vi "Input Quantities.vi"() -> ()   [LabVIEW 2013]
uses:
  qwtblvlib/TD Quantity.ctl
  TD Input Quantities qeue values.ctl
  <vilib>/Analysis/Matrix/Datatypes/RealMatrix.ctl
  globals.vi
  <vilib>/Utility/xml.llb/Write to XML File(string).vi
  <vilib>/Utility/xml.llb/Read From XML File(string).vi
  <vilib>/Utility/file.llb/Read From Spreadsheet File (DBL).vi
  <vilib>/Analysis/Matrix/Numeric/Conversions/Matrix To Array - RM.vi
  <vilib>/Analysis/Matrix/NI_Matrix.lvlib
  qwtblvlib/QWTBLVLib.lvlib
panel:
  in  "qeue cases":T1=enum."update list of quantities"
  out "current Q index":i32 min=0
  in  "r-randomize":bool
  in  "corr-default":bool
  in  "dof-fill":bool
  in  "uncertainty-fill":bool
  in  "value-load CSV":bool
  in  "hide this panel":bool
  in  "import data":bool
  in  "generate wvfrm":bool
  in  "Q":T2={"Name"="", "Value"=[[1.0]], "Uncertainty"=[[1.0]], "Degrees of Freedom"=[[10.0]], "Correlation"=[[10.0]], "Randomized uncertainty"=[[10.0]]} caption="Selected Quantity"
  in  "load all":bool
  in  "save all":bool
  in  "Q list":i32(listbox) caption="List of\nInput Quantities"
  in  "remove Q":bool
  in  "add Q":bool
  in  "rand-clear":bool
  in  "corr-clear":bool
  in  "dof-clear":bool
  in  "uncertainty-clear":bool
  in  "value-clear":bool
  # "Input Quantities"
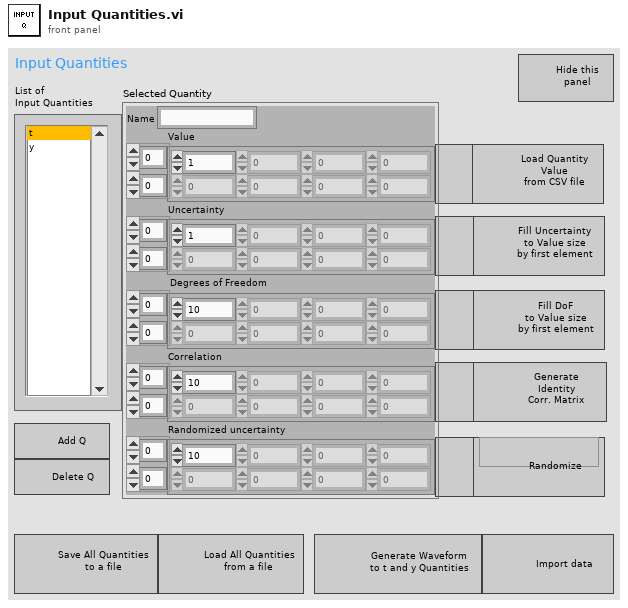
[diagram p1: front panel]
types:
  T1 = typedef "TD Input Quantities qeue values.ctl" = enum16{"hide VI", "current Q to datain", "update list of quantities", "show current quantity", "quit"}
  T2 = typedef "QWTBLVLib.lvlib/TD Quantity.ctl" = cluster{"Name":string, "Value":dbl[][], "Uncertainty":dbl[][], "Degrees of Freedom":dbl[][], "Correlation":dbl[][], "Randomized uncertainty":dbl[][]}
  T3 = enum32{"Invalid", "Standard", "Closed", "Hidden", "Minimized", "Maximized"}
  T4 = enum8{"Enabled", "Disabled", "Disabled and Grayed Out"}
  T5 = cluster{"Name":string, "Value":dbl[][], "Uncertainty":dbl[][], "Degrees of\nFreedom":dbl[][], "Correlation":dbl[][], "Randomized uncertainty":dbl[][]}
  T6 = typedef "NI_Matrix.lvlib/RealMatrix.ctl" = dbl[][]
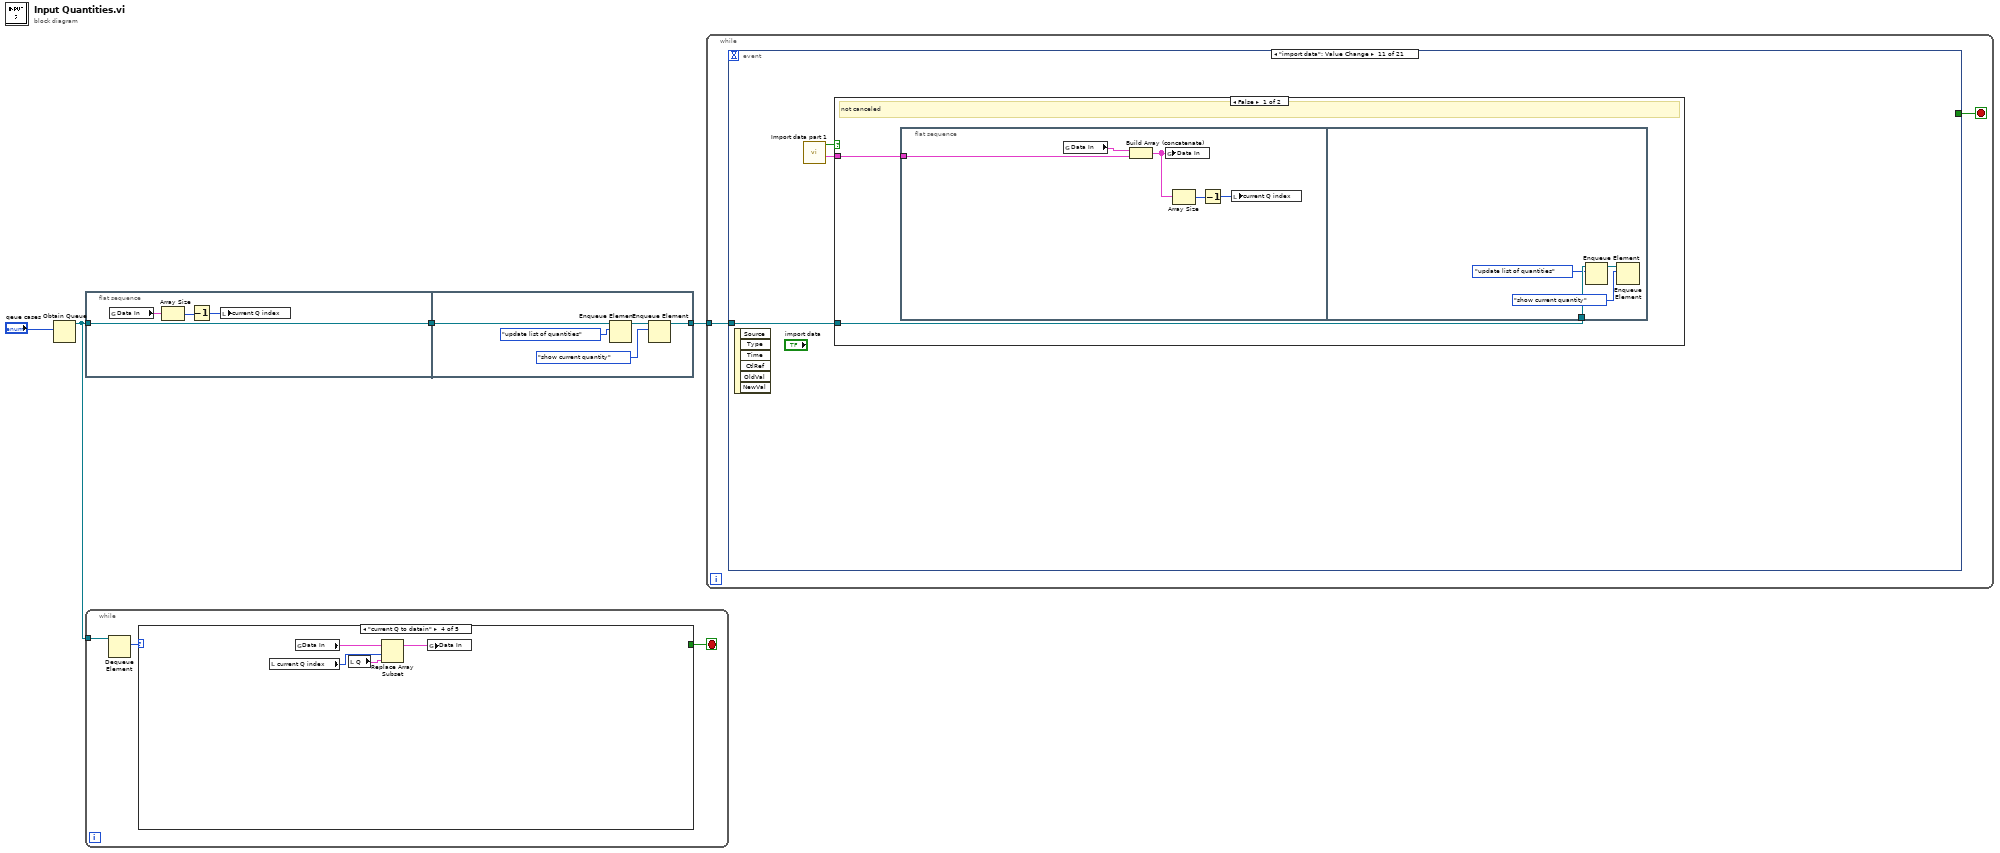
[diagram p0: block diagram]
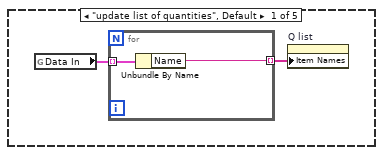
[diagram p2: hidden frame]
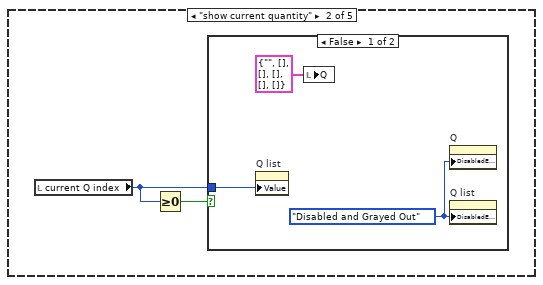
[diagram p3: hidden frame]
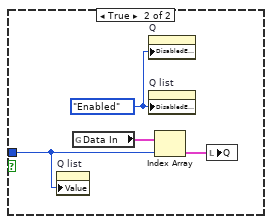
[diagram p4: hidden frame]
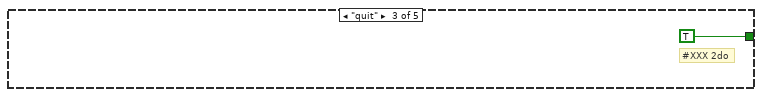
[diagram p5: hidden frame]
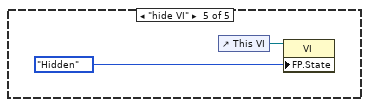
[diagram p6: hidden frame]
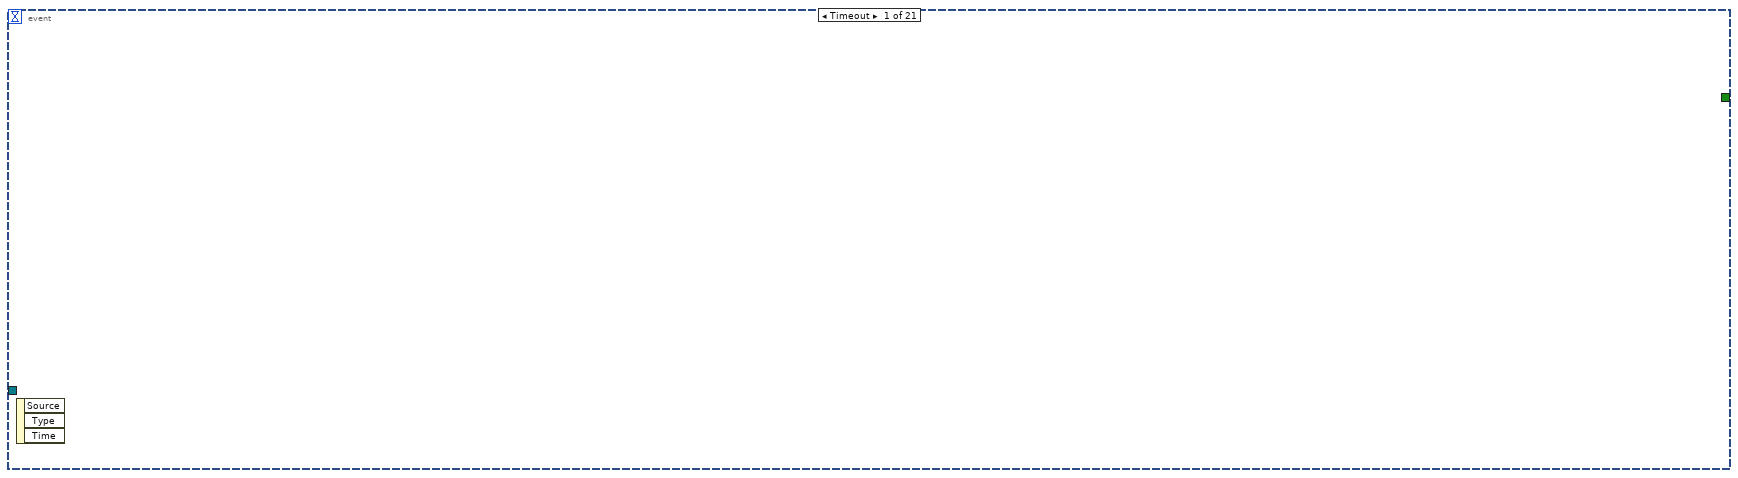
[diagram p7: hidden frame]
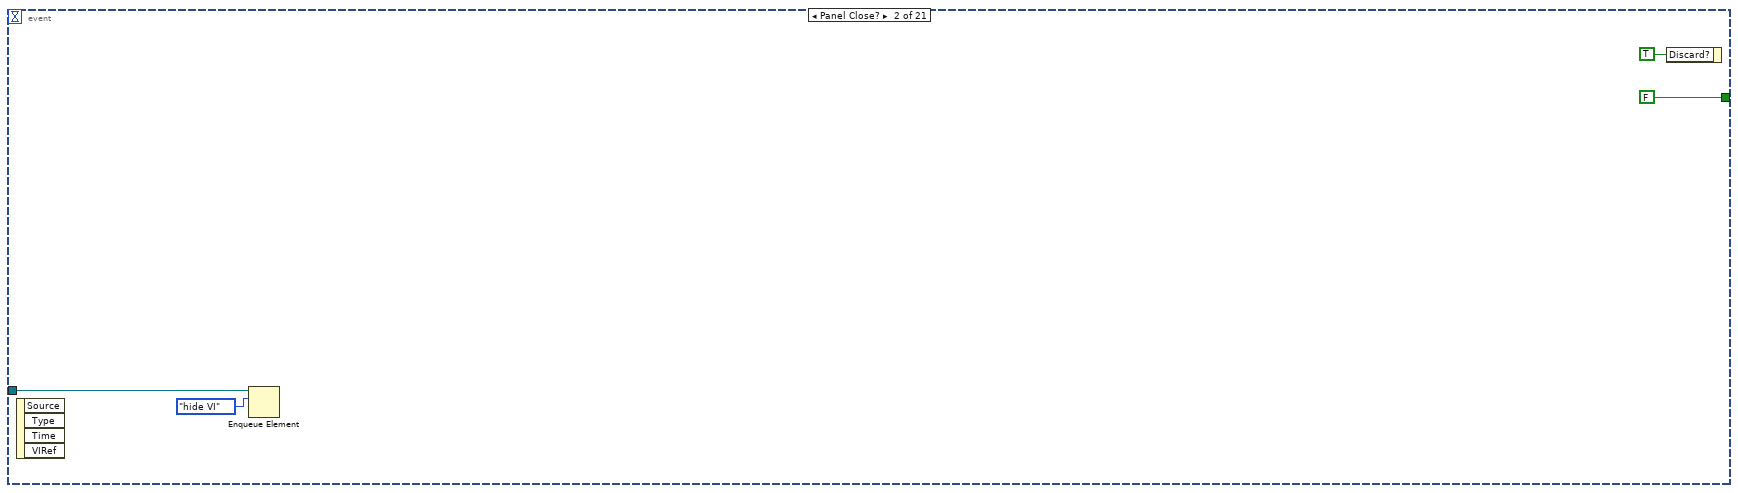
[diagram p8: hidden frame]
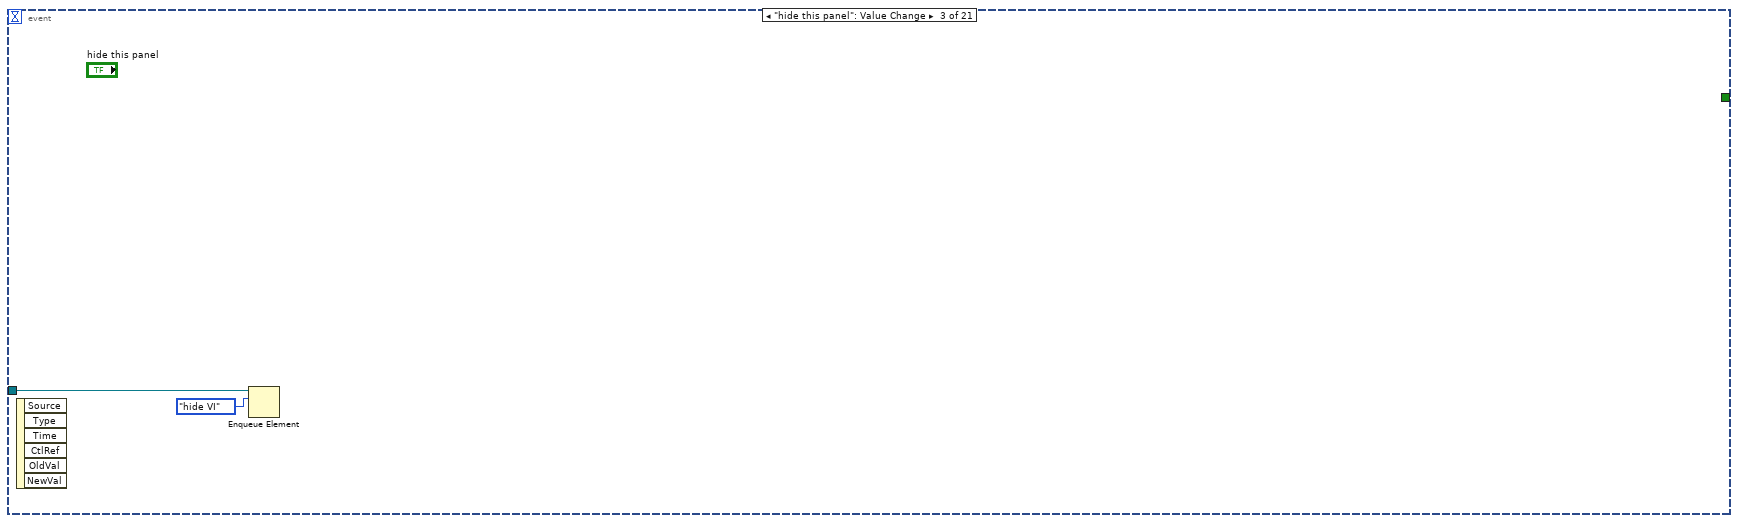
[diagram p9: hidden frame]
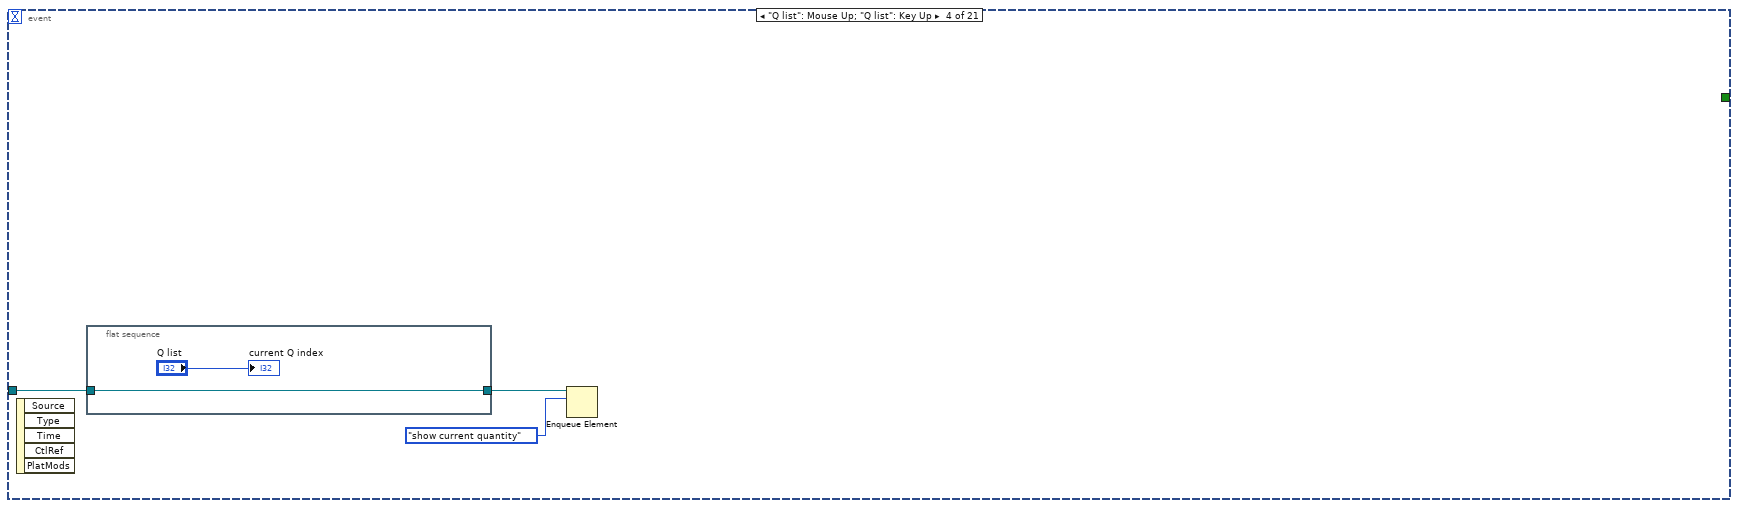
[diagram p10: hidden frame]
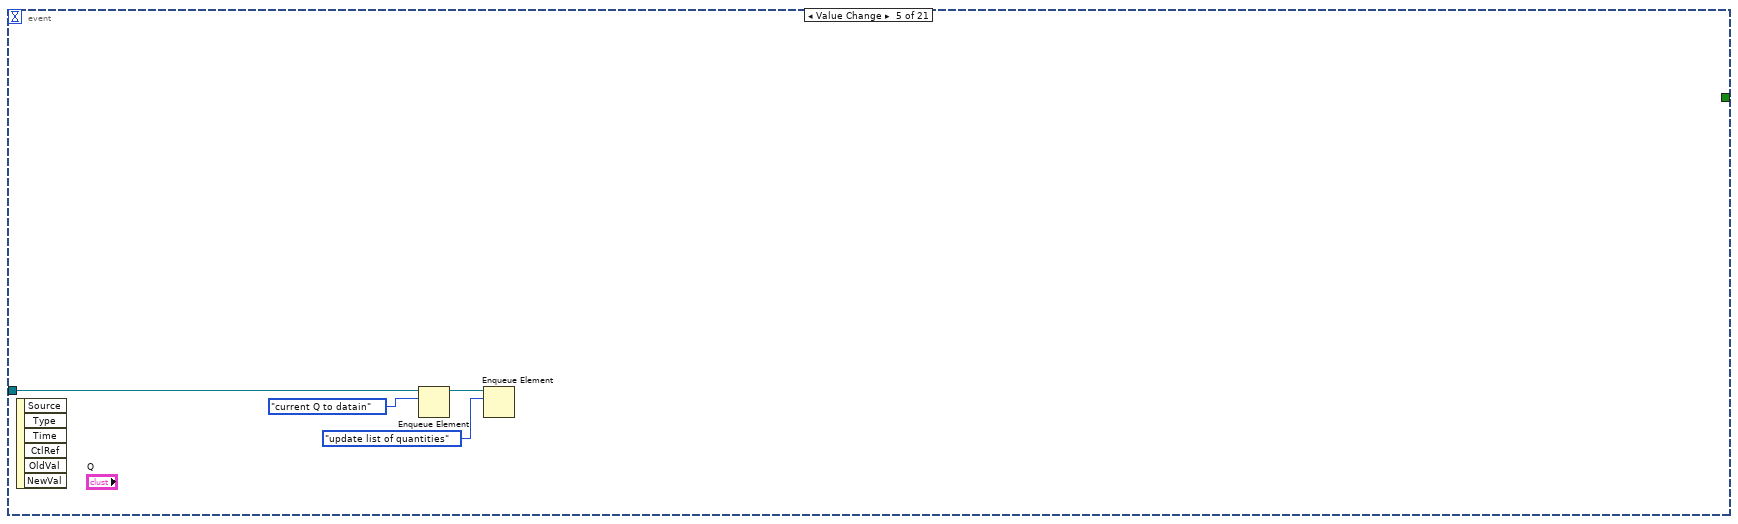
[diagram p11: hidden frame]
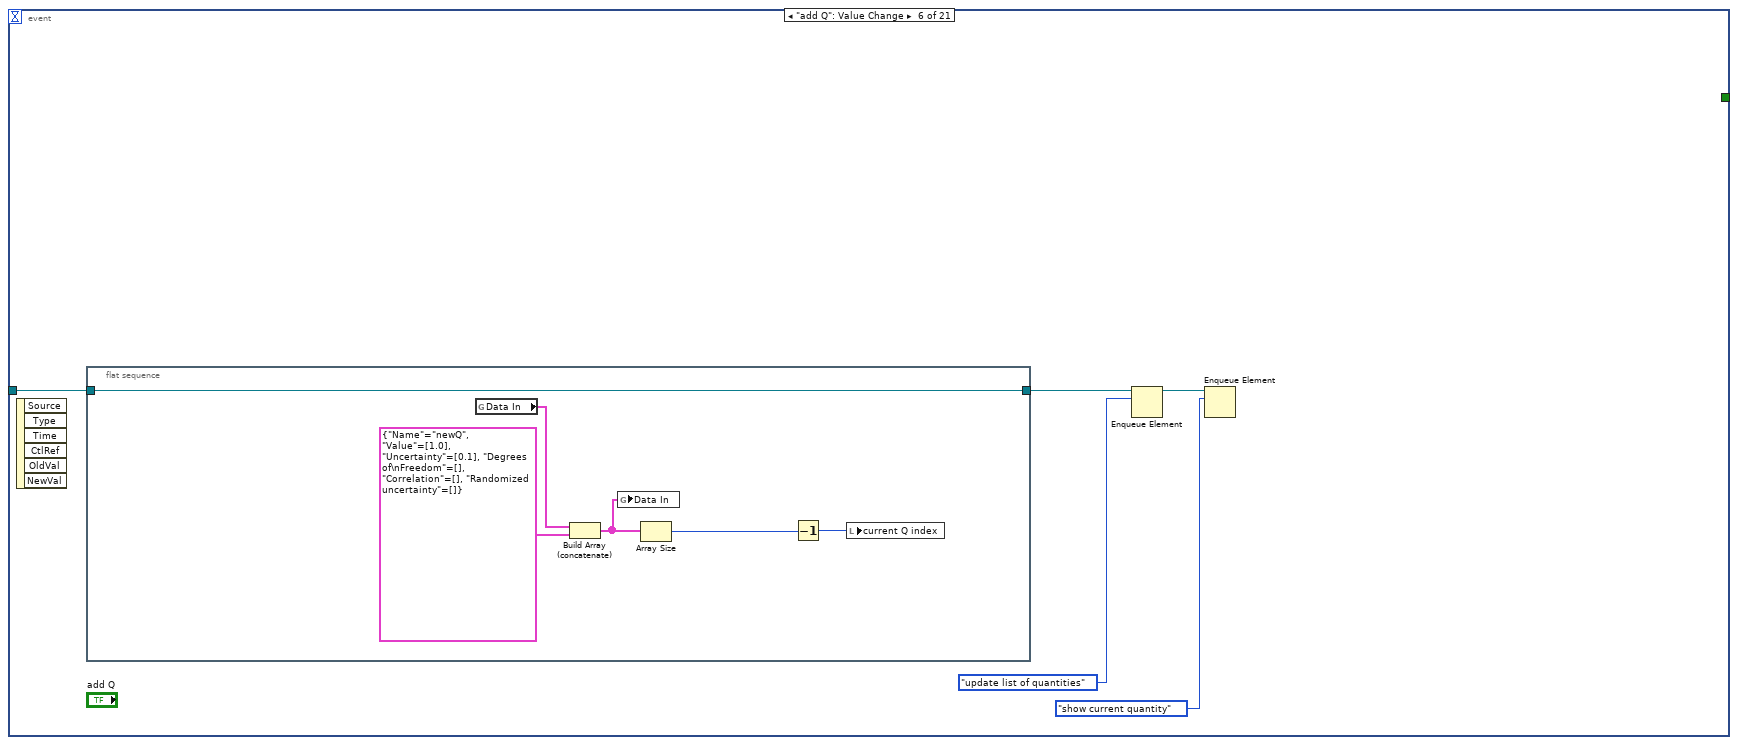
[diagram p12: hidden frame]
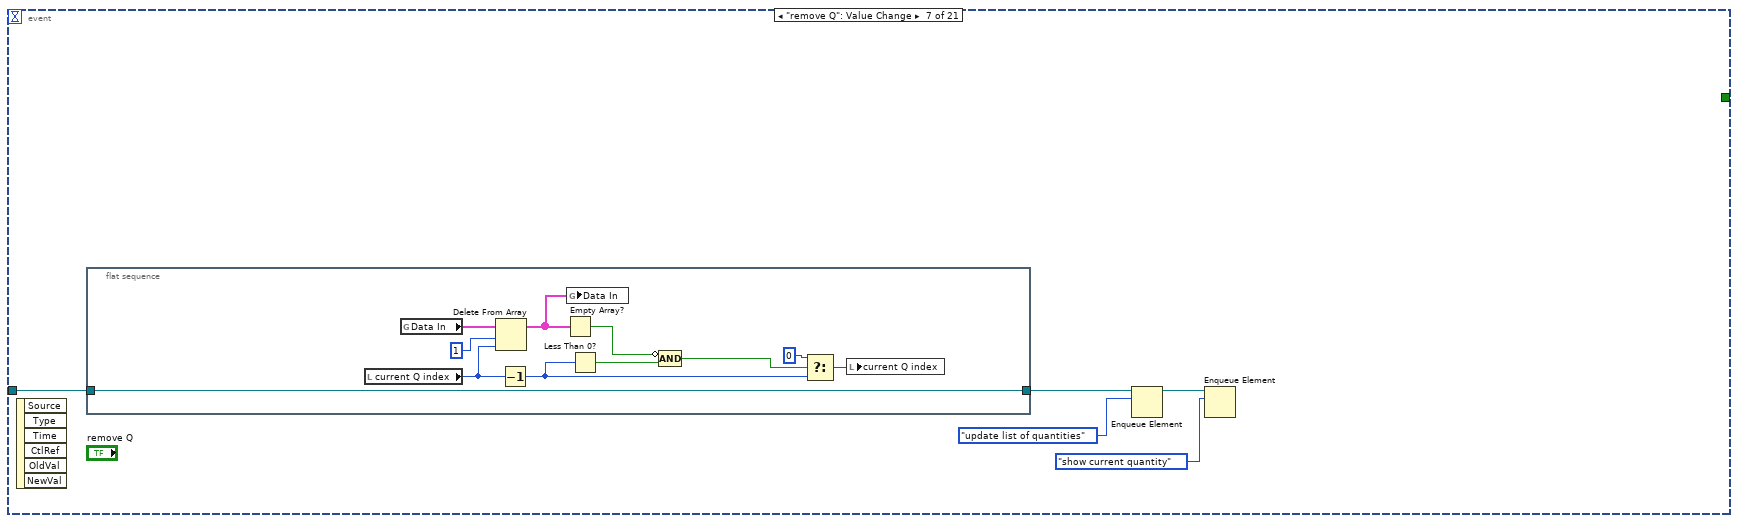
[diagram p13: hidden frame]
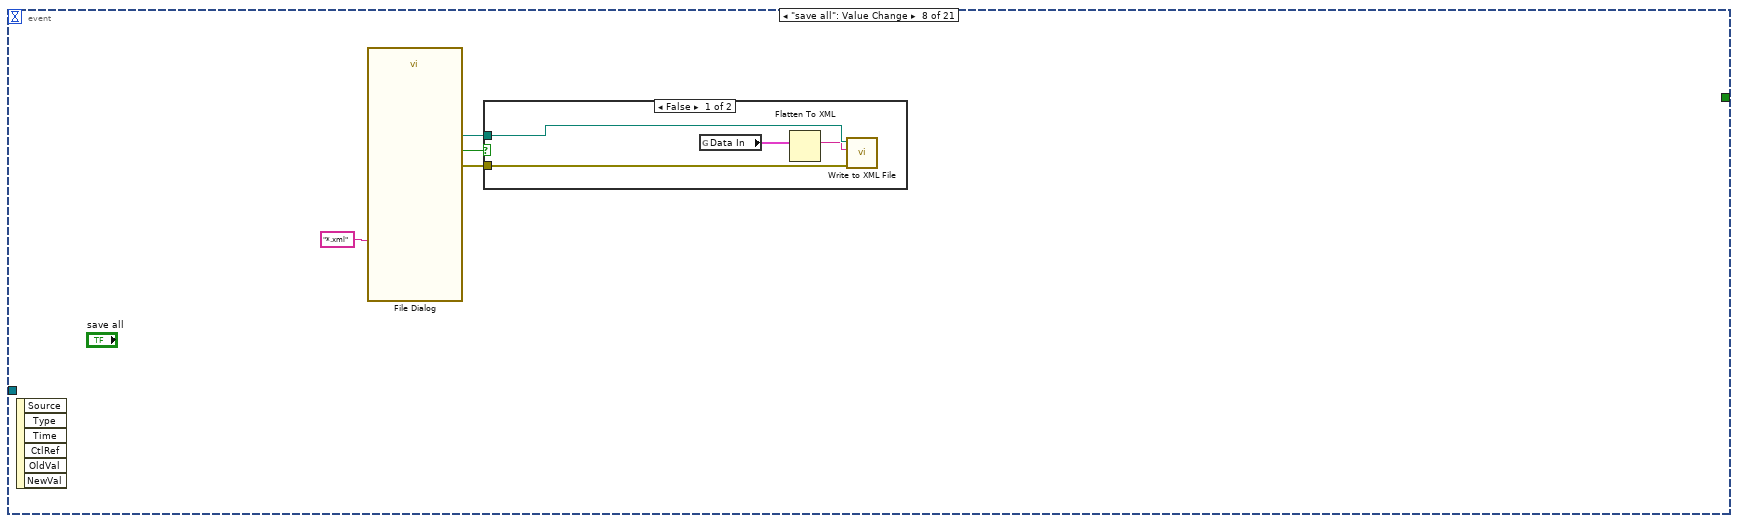
[diagram p14: hidden frame]
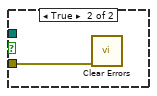
[diagram p15: hidden frame]
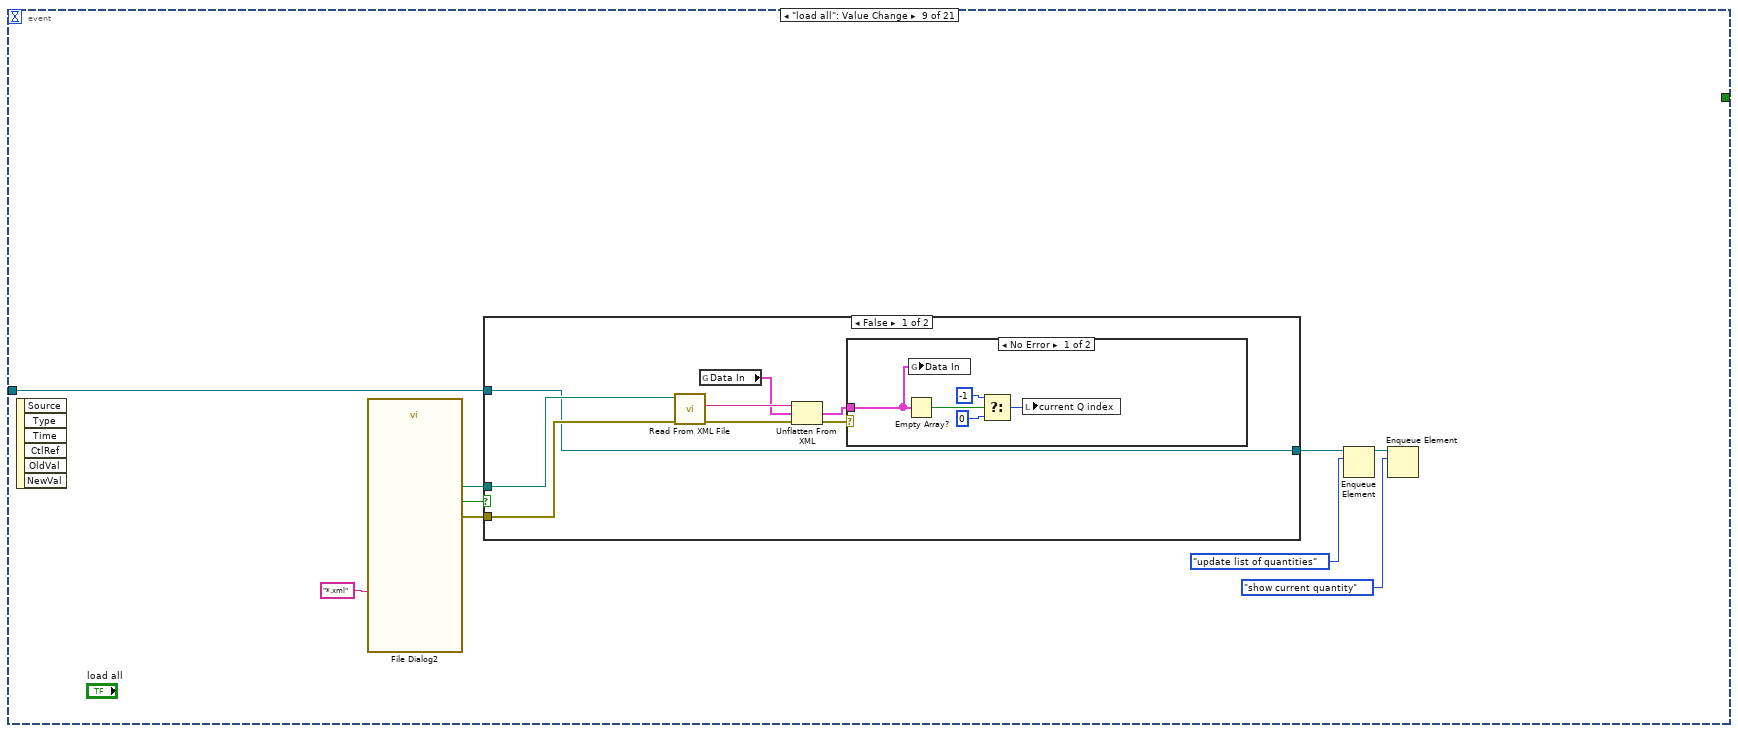
[diagram p16: hidden frame]
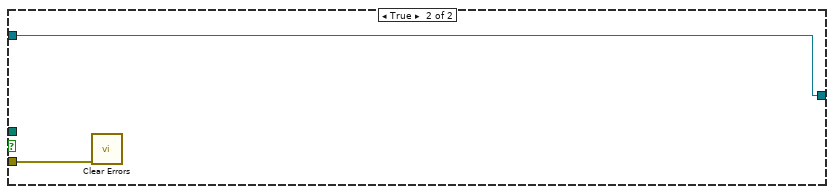
[diagram p18: hidden frame]
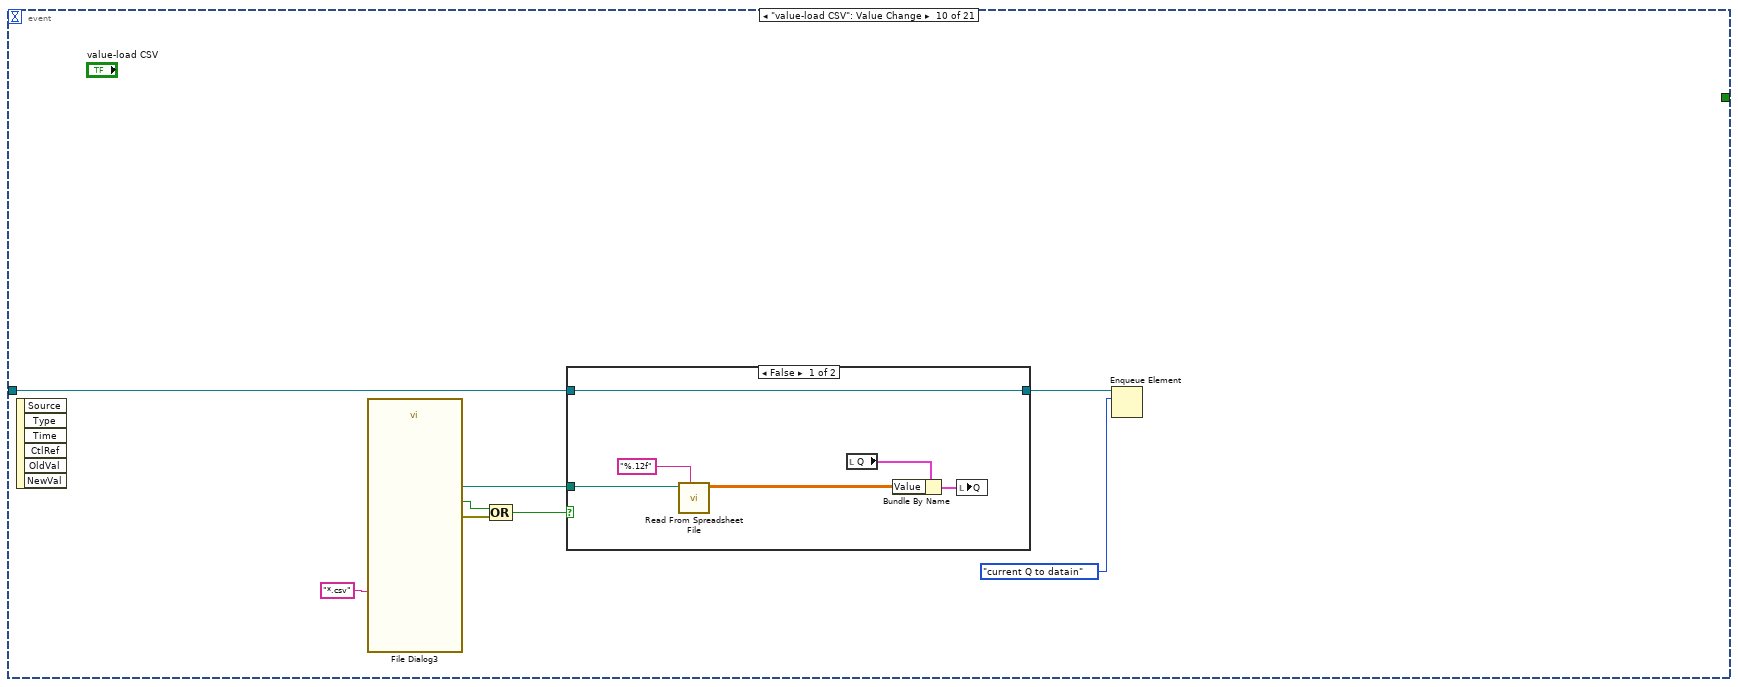
[diagram p19: hidden frame]
diagram:
  n1 = Obtain Queue(element data type="qeue cases") -> (queue out=w3:refnum<queue>)  [unwired: 4 in, 2 out]
  n2 = flat-sequence {
    tunnel: w3 -> [w8]
    tunnel: [w8] -> w1
    tunnel: [w9] -> w2
    tunnel: w1 -> [w13]
    frame #0 {
      n3 = global read "globals.vi" "Data In"() -> (w7:T2[])
      n4 = Array Size(array=w7) -> (size(s)=w6:i32)
      n5 = Decrement(x=w6) -> (x-1=w5:i32)
      n6 = local write "current Q index"(w5) -> ()
    }
    frame #1 {
      n7 = Enqueue Element(queue=w13, element=TD_Input_Quantities_qeue_values."update list of quantities") -> (queue out=w11:refnum<queue>)  [unwired: 2 in, 2 out]
      n8 = Enqueue Element(queue=w11, element=TD_Input_Quantities_qeue_values."show current quantity") -> (queue out=w9:refnum<queue>)  [unwired: 2 in, 2 out]
    }
  }
  n9 = while {
    tunnel: w3 -> [w16]
    stop <- w14 stop-if-true
    n10 = Dequeue Element(queue=w16) -> (element=w15:T1)  [unwired: 2 in, 3 out]
    n11 = case shown="\"current Q to datain\"" w15 {
      tunnel: [_ _ TRUE _ _] -> w14
      frame "update list of quantities", Default {
        n12 = global read "globals.vi" "Data In"() -> (w17:T2[])
        n13 = for {
          tunnel: [w20] -> w18 mode=indexing
          tunnel: w17 -> [w19] mode=indexing
          n14 = Unbundle By Name(w19) -> ("Name"=w20:string)
        }
        n15 = property on="Q list" class="LstBox (strict)"("Item Names"=w18) -> ()  [unwired: 2 in, 2 out]
      }
      frame "show current quantity" {
        n16 = local read "current Q index"() -> (w22:i32)
        n17 = Greater Or Equal To 0?(x=w22) -> (x >= 0?=w21:bool)
        n18 = case shown="False" w21 {
          tunnel: w22 -> [w24 w27]
          frame False {
            w23 = T4."Disabled and Grayed Out" ("Disabled")
            n19 = property on="Q list" class="LstBox (strict)"("Value"=w24) -> ()  [unwired: 2 in, 2 out]
            n20 = local write "Q"(T2 {"Name"="", "Value"=[], "Uncertainty"=[], "Degrees of Freedom"=[], "Correlation"=[], "Randomized uncertainty"=[]} ("Q")) -> ()
            n21 = property on="Q" class="Clust (strict)"("DisabledEnum"=w23) -> ()  [unwired: 2 in, 2 out]
            n22 = property on="Q list" class="LstBox (strict)"("DisabledEnum"=w23) -> ()  [unwired: 2 in, 2 out]
          }
          frame True {
            w26 = T4."Enabled" ("Disabled")
            n23 = property on="Q list" class="LstBox (strict)"("Value"=w27) -> ()  [unwired: 2 in, 2 out]
            n24 = global read "globals.vi" "Data In"() -> (w28:T2[])
            n25 = property on="Q" class="Clust (strict)"("DisabledEnum"=w26) -> ()  [unwired: 2 in, 2 out]
            n26 = property on="Q list" class="LstBox (strict)"("DisabledEnum"=w26) -> ()  [unwired: 2 in, 2 out]
            n27 = Index Array(array=w28, index=w27) -> (element=w29:T2)
            n28 = local write "Q"(w29) -> ()
          }
        }
      }
      frame "quit" {
        # "#XXX 2do"
      }
      frame "current Q to datain" {
        n29 = local read "current Q index"() -> (w34:i32)
        n30 = global read "globals.vi" "Data In"() -> (w32:T2[])
        n31 = local read "Q"() -> (w31:T2)
        n32 = Replace Array Subset(array=w32, new element=w31, index=w34) -> (w33:T2[])
        n33 = global write "globals.vi" "Data In"(w33) -> ()
      }
      frame "hide VI" {
        n34 = control-ref of="This VI"() -> (w35:refnum<vi>)
        n35 = property class="VI"(reference=w35, "FP.State"=T3."Hidden" ("Front Panel Window:State")) -> ()  [unwired: 1 in, 2 out]
      }
    }
  }
  n36 = while {
    tunnel: w2 -> [w37]
    stop <- w38 stop-if-true
    n37 = event shown="[10] \"import data\": Value Change" {
      selector: _ -> [_ _ _ _ _ _ _ _ _ _ _ _ _ _ _ _ _ _ _ _ _]
      dyn-events: _ -> [_ _ _ _ _ _ _ _ _ _ _ _ _ _ _ _ _ _ _ _ _]
      timeout: _ -> [_ _ _ _ _ _ _ _ _ _ _ _ _ _ _ _ _ _ _ _ _]
      tunnel: [_ FALSE _ _ _ _ _ _ _ _ _ _ _ _ _ _ _ _ _ _ _] -> w38
      tunnel: w37 -> [_ w40 w43 w46 w50 w55 w66 _ w94 w119 w131 w145 w162 w178 w207 w250 w257 w263 w271 w278 w291]
      event Timeout {
        n38 = event-data() -> ()  [unwired: 1 in, 3 out]
      }
      event Panel Close? {
        n39 = event-data() -> ()  [unwired: 1 in, 4 out]
        n40 = Enqueue Element(queue=w40, element=TD_Input_Quantities_qeue_values."hide VI") -> ()  [unwired: 2 in, 3 out]
        n41 = event-data("Discard?"=TRUE) -> ()  [unwired: 1 in, 1 out]
      }
      event "hide this panel": Value Change {
        n42 = event-data() -> ()  [unwired: 1 in, 6 out]
        n43 = Enqueue Element(queue=w43, element=TD_Input_Quantities_qeue_values."hide VI") -> ()  [unwired: 2 in, 3 out]
      }
      event "Q list": Mouse Up; "Q list": Key Up {
        n44 = event-data() -> ()  [unwired: 1 in, 5 out]
        n45 = flat-sequence {
          tunnel: [w49] -> w45
          tunnel: w46 -> [w49]
          frame #0 {
            "current Q index" <- "Q list"
          }
        }
        n46 = Enqueue Element(queue=w45, element=TD_Input_Quantities_qeue_values."show current quantity") -> ()  [unwired: 2 in, 3 out]
      }
      event Value Change {
        n47 = event-data() -> ()  [unwired: 1 in, 6 out]
        n48 = Enqueue Element(queue=w50, element=TD_Input_Quantities_qeue_values."current Q to datain") -> (queue out=w52:refnum<queue>)  [unwired: 2 in, 2 out]
        n49 = Enqueue Element(queue=w52, element=TD_Input_Quantities_qeue_values."update list of quantities") -> ()  [unwired: 2 in, 3 out]
      }
      event "add Q": Value Change {
        n50 = event-data() -> ()  [unwired: 1 in, 6 out]
        n51 = flat-sequence {
          tunnel: [w59] -> w54
          tunnel: w55 -> [w59]
          frame #0 {
            n52 = global read "globals.vi" "Data In"() -> (w62:T2[])
            n53 = Build Array (concatenate)(w62, T5 {"Name"="newQ", "Value"=[[1.0]], "Uncertainty"=[[0.1]], "Degrees of\nFreedom"=[], "Correlation"=[], "Randomized uncertainty"=[]} ("Quantity")) -> (w61:T2[])
            n54 = global write "globals.vi" "Data In"(w61) -> ()
            n55 = Array Size(array=w61) -> (size(s)=w64:i32)
            n56 = Decrement(x=w64) -> (x-1=w60:i32)
            n57 = local write "current Q index"(w60) -> ()
          }
        }
        n58 = Enqueue Element(queue=w54, element=TD_Input_Quantities_qeue_values."update list of quantities") -> (queue out=w58:refnum<queue>)  [unwired: 2 in, 2 out]
        n59 = Enqueue Element(queue=w58, element=TD_Input_Quantities_qeue_values."show current quantity") -> ()  [unwired: 2 in, 3 out]
      }
      event "remove Q": Value Change {
        n60 = event-data() -> ()  [unwired: 1 in, 6 out]
        n61 = flat-sequence {
          tunnel: w66 -> [w70]
          tunnel: [w70] -> w65
          frame #0 {
            n62 = local read "current Q index"() -> (w71:i32)
            n63 = global read "globals.vi" "Data In"() -> (w72:T2[])
            n64 = Delete From Array(array=w72, length=1, index=w71) -> (array with subset deleted=w74:T2[])  [unwired: 1 out]
            n65 = Decrement(x=w71) -> (x-1=w79:i32)
            n66 = Empty Array?(array=w74) -> (empty?=w75:bool)
            n67 = global write "globals.vi" "Data In"(w74) -> ()
            n68 = Less Than 0?(x=w79) -> (x < 0?=w77:bool)
            n69 = Compound Arithmetic op=AND(invert w75, w77) -> (w78:bool)
            n70 = Select(t=0, s=w78, f=w79) -> (s? t:f=w80:i32)
            n71 = local write "current Q index"(w80) -> ()
          }
        }
        n72 = Enqueue Element(queue=w65, element=TD_Input_Quantities_qeue_values."update list of quantities") -> (queue out=w68:refnum<queue>)  [unwired: 2 in, 2 out]
        n73 = Enqueue Element(queue=w68, element=TD_Input_Quantities_qeue_values."show current quantity") -> ()  [unwired: 2 in, 3 out]
      }
      event "save all": Value Change {
        n74 = event-data() -> ()  [unwired: 1 in, 6 out]
        n75 = call "File Dialog"("pattern (all files)"="*.xml") -> ("selected path"=w84:path, "cancelled"=w82:bool, "error out"=w83:errorcluster)  [unwired: 11 in, 1 out]
        n76 = case shown="False" w82 {
          tunnel: w83 -> [w87 w89]
          tunnel: w84 -> [w88 _]
          frame False {
            n77 = global read "globals.vi" "Data In"() -> (w85:T2[])
            n78 = Flatten To XML(anything=w85) -> (xml string=w86:string)
            n79 = call-poly <vilib>:"Write to XML File.vi"("error in (no error)"=w87, "XML Input"=w86, "XML File Path"=w88) -> ()  [unwired: 6 in, 3 out]
          }
          frame True {
            n80 = call <vilib>:"Clear Errors.vi"("error in (no error)"=w89) -> ()  [unwired: 6 in, 1 out]
          }
        }
      }
      event "load all": Value Change {
        n81 = event-data() -> ()  [unwired: 1 in, 6 out]
        n82 = call "File Dialog2"("pattern (all files)"="*.xml") -> ("selected path"=w98:path, "cancelled"=w96:bool, "error out"=w97:errorcluster)  [unwired: 11 in, 1 out]
        n83 = case shown="False" w96 {
          tunnel: w97 -> [w105 w113]
          tunnel: w98 -> [w106 _]
          tunnel: w94 -> [w99 w112]
          tunnel: [w99 w112] -> w90
          frame False {
            n84 = call-poly <vilib>:"Read From XML File.vi"("error in (no error)"=w105, "XML File Path"=w106) -> ("error out"=w103:errorcluster, "XML Elements"=w104:string)  [unwired: 7 in, 1 out]
            n85 = global read "globals.vi" "Data In"() -> (w100:T2[])
            n86 = Unflatten From XML(xml string=w104, type=w100, error in (no error)=w103) -> (value=w101:T2[], error out=w102:errorcluster)
            n87 = case shown="No Error" w102 {
              tunnel: w101 -> [w111 _]
              frame No Error {
                n88 = Empty Array?(array=w111) -> (empty?=w110:bool)
                n89 = global write "globals.vi" "Data In"(w111) -> ()
                n90 = Select(t=-1, s=w110, f=0 ("current Q index")) -> (s? t:f=w108:i32)
                n91 = local write "current Q index"(w108) -> ()
              }
              frame Error {
              }
            }
          }
          frame True {
            n92 = call <vilib>:"Clear Errors.vi"("error in (no error)"=w113) -> ()  [unwired: 6 in, 1 out]
          }
        }
        n93 = Enqueue Element(queue=w90, element=TD_Input_Quantities_qeue_values."update list of quantities") -> (queue out=w91:refnum<queue>)  [unwired: 2 in, 2 out]
        n94 = Enqueue Element(queue=w91, element=TD_Input_Quantities_qeue_values."show current quantity") -> ()  [unwired: 2 in, 3 out]
      }
      event "value-load CSV": Value Change {
        n95 = event-data() -> ()  [unwired: 1 in, 6 out]
        n96 = call "File Dialog3"("pattern (all files)"="*.csv") -> ("selected path"=w120:path, "cancelled"=w118:bool, "error out"=w117:errorcluster)  [unwired: 11 in, 1 out]
        n97 = Compound Arithmetic op=OR(w118, w117) -> (w116:bool)
        n98 = case shown="False" w116 {
          tunnel: w120 -> [w127 _]
          tunnel: w119 -> [w122 w128]
          tunnel: [w122 w128] -> w114
          frame False {
            n99 = call-poly <vilib>:"Read From Spreadsheet File.vi"("format (%.3f)"="%.12f", "file path (dialog if empty)"=w127) -> ("all rows"=w125:dbl[][])  [unwired: 5 in, 4 out]
            n100 = local read "Q"() -> (w126:T2)
            n101 = Bundle By Name(cluster=w126, "Value"=w125) -> (w124:T2)
            n102 = local write "Q"(w124) -> ()
          }
          frame True {
          }
        }
        n103 = Enqueue Element(queue=w114, element=TD_Input_Quantities_qeue_values."current Q to datain") -> ()  [unwired: 2 in, 3 out]
      }
      event "import data": Value Change {
        n104 = event-data() -> ()  [unwired: 1 in, 6 out]
        n105 = call "Import data part 1.vi"() -> ("New Qs"=w129:T2[], "canceled?"=w130:bool)  [unwired: 10 in]
        n106 = case shown="False" w130 {
          tunnel: w131 -> [w133 _]
          tunnel: w129 -> [w132 _]
          frame False {
            # "not canceled"
            n107 = flat-sequence {
              tunnel: w132 -> [w137]
              tunnel: w133 -> [w142]
              frame #0 {
                n108 = global read "globals.vi" "Data In"() -> (w138:T2[])
                n109 = Build Array (concatenate)(w138, w137) -> (w135:T2[])
                n110 = global write "globals.vi" "Data In"(w135) -> ()
                n111 = Array Size(array=w135) -> (size(s)=w134:i32)
                n112 = Decrement(x=w134) -> (x-1=w136:i32)
                n113 = local write "current Q index"(w136) -> ()
              }
              frame #1 {
                n114 = Enqueue Element(queue=w142, element=TD_Input_Quantities_qeue_values."update list of quantities") -> (queue out=w139:refnum<queue>)  [unwired: 2 in, 2 out]
                n115 = Enqueue Element(queue=w139, element=TD_Input_Quantities_qeue_values."show current quantity") -> ()  [unwired: 2 in, 3 out]
              }
            }
          }
          frame True {
            # "canceled"
          }
        }
      }
      event "uncertainty-fill": Value Change {
        n116 = event-data() -> ()  [unwired: 1 in, 6 out]
        n117 = flat-sequence {
          tunnel: w145 -> [w146]
          tunnel: [w146] -> w144
          frame #0 {
            n118 = local read "Q"() -> (w159:T2)
            n119 = Unbundle By Name(w159) -> ("Value"=w157:dbl[][], "Uncertainty"=w147:dbl[][])
            n120 = Array Size(array=w157) -> (size(s)=w153:i32[])
            n121 = Index Array(array=w147, index (row)=0, index (col)=0 ("disabled index (col)")) -> (element=w154:dbl)
            n122 = Index Array(array=w153, index #1=0 ("index"), index #2=1 ("index")) -> (element #1=w150:i32, element #2=w149:i32)
            n123 = Initialize Array(w154, w150, w149) -> (w148:dbl[][])
            n124 = Bundle By Name(cluster=w159, "Uncertainty"=w148) -> (w158:T2)
            n125 = local write "Q"(w158) -> ()
          }
        }
        n126 = Enqueue Element(queue=w144, element=TD_Input_Quantities_qeue_values."current Q to datain") -> ()  [unwired: 2 in, 3 out]
      }
      event "dof-fill": Value Change {
        n127 = event-data() -> ()  [unwired: 1 in, 6 out]
        n128 = flat-sequence {
          tunnel: w162 -> [w163]
          tunnel: [w163] -> w161
          frame #0 {
            n129 = local read "Q"() -> (w176:T2)
            n130 = Unbundle By Name(w176) -> ("Value"=w174:dbl[][], "Degrees of Freedom"=w164:dbl[][])
            n131 = Array Size(array=w174) -> (size(s)=w170:i32[])
            n132 = Index Array(array=w164, index (row)=0, index (col)=0 ("disabled index (col)")) -> (element=w171:dbl)
            n133 = Index Array(array=w170, index #1=0 ("index"), index #2=1 ("index")) -> (element #1=w167:i32, element #2=w166:i32)
            n134 = Initialize Array(w171, w167, w166) -> (w165:dbl[][])
            n135 = Bundle By Name(cluster=w176, "Degrees of Freedom"=w165) -> (w175:T2)
            n136 = local write "Q"(w175) -> ()
          }
        }
        n137 = Enqueue Element(queue=w161, element=TD_Input_Quantities_qeue_values."current Q to datain") -> ()  [unwired: 2 in, 3 out]
      }
      event "corr-default": Value Change {
        n138 = event-data() -> ()  [unwired: 1 in, 6 out]
        n139 = flat-sequence {
          tunnel: w178 -> [w180]
          tunnel: [w180] -> w177
          frame #0 {
            n140 = local read "Q"() -> (w187:T2)
            n141 = Unbundle By Name(w187) -> ("Value"=w185:dbl[][])
            n142 = call "Scalar Vector Matrix in 2D.vi"("2D Array"=w185) -> ("Is Matrix?"=w184:bool, "Is Empty?"=w181:bool, "Dim Max"=w182:i32, "Dimensions"=w183:i32[])  [unwired: 4 in, 3 out]
            n143 = case shown="False" w181 {
              tunnel: w187 -> [w192 w206]
              tunnel: [w191 w205] -> w186
              tunnel: w184 -> [w190 _]
              tunnel: w183 -> [w189 _]
              tunnel: w182 -> [w188 _]
              frame False {
                # "vector or matrix"
                n144 = case shown="False" w190 {
                  tunnel: w192 -> [w202 w203]
                  tunnel: [w201 w203] -> w191
                  tunnel: w189 -> [_ _]
                  tunnel: w188 -> [w193 _]
                  frame False {
                    # "vector"
                    n145 = Resize Matrix(1:w193, 2:w193, 4:T6 [] ("matrix")) -> (0:w196:T6)
                    n146 = Replace Array Subset(array=w196, new element=1.0 ("new diagonal/fill element"), index (row)=0 ("disabled index (row)"), index (col)=0 ("disabled index (col)")) -> (w195:T6)
                    n147 = call-poly <vilib>:"Matrix To Array.vi"("Real Matrix"=w195) -> ("Real 2D Array"=w194:dbl[][])
                    n148 = Bundle By Name(cluster=w202, "Correlation"=w194) -> (w201:T2)
                  }
                  frame True {
                    # "matrix"
                  }
                }
              }
              frame True {
                # "empty array"
                n149 = Bundle By Name(cluster=w206, "Correlation"=dbl[][] []) -> (w205:T2)
              }
            }
            n150 = local write "Q"(w186) -> ()
          }
        }
        n151 = Enqueue Element(queue=w177, element=TD_Input_Quantities_qeue_values."current Q to datain") -> ()  [unwired: 2 in, 3 out]
      }
      event "r-randomize": Value Change {
        # "#2do"
        n152 = event-data() -> ()  [unwired: 1 in, 6 out]
        n153 = local read "Q"() -> (w214:T2)
        n154 = Unbundle By Name(w214) -> ("Value"=w218:dbl[][], "Uncertainty"=w212:dbl[][])
        n155 = call "Scalar Vector Matrix in 2D.vi"("2D Array"=w218) -> ("Is Matrix?"=w217:bool, "Is Vector?"=w213:bool, "Is Empty?"=w215:bool, "Dim Max"=w211:i32, "Dim Min"=w210:i32)  [unwired: 4 in, 2 out]
        n156 = Or(x=w215, y=w217) -> (x .or. y?=w216:bool)
        n157 = case shown="True" w216 {
          tunnel: w215 -> [_ w244]
          tunnel: w214 -> [w235 w243]
          tunnel: w213 -> [_ _]
          tunnel: w212 -> [w234 _]
          tunnel: w211 -> [w233 _]
          tunnel: w210 -> [w231 _]
          tunnel: [w226 w243] -> w209
          tunnel: [w225 TRUE ("Canceled?")] -> w208
          frame False {
            n158 = call "Scalar Vector Matrix in 2D.vi"("2D Array"=w234) -> ("Dim Max"=w232:i32, "Dim Min"=w230:i32)  [unwired: 4 in, 5 out]
            n159 = Equal?(x=w233, y=w232) -> (x = y?=w228:bool)
            n160 = Equal?(x=w231, y=w230) -> (x = y?=w229:bool)
            n161 = And(x=w228, y=w229) -> (x .and. y?=w227:bool)
            n162 = case shown="False" w227 {
              tunnel: w235 -> [w237 w241]
              tunnel: [w237 w240] -> w226
              tunnel: [TRUE ("Canceled?") w239] -> w225
              frame False {
                n163 = One Button Dialog(message="Values and uncertainties of Quantity\nhas different dimensions.") -> ()  [unwired: 1 in, 1 out]
              }
              frame True {
                n164 = call "Randomize.vi"("Quantity"=w241) -> ("Canceled?"=w239:bool, "Randomized Quantity"=w240:T2)  [unwired: 9 in]
              }
            }
          }
          frame True {
            n165 = case shown="False" w244 {
              frame False {
                n166 = One Button Dialog(message="Cannot do for matrix quantity.\nImplemented only for scalars or vectors.", button name ("OK")="OK") -> ()  [unwired: 1 out]
              }
              frame True {
                n167 = One Button Dialog(message="Value matrix is empty!", button name ("OK")="OK") -> ()  [unwired: 1 out]
              }
            }
          }
        }
        n168 = case shown="False" w208 {
          tunnel: w209 -> [w222 _]
          tunnel: w207 -> [w220 _]
          frame False {
            n169 = flat-sequence {
              tunnel: w222 -> [w224]
              tunnel: w220 -> [w223]
              tunnel: [w223] -> w219
              frame #0 {
                n170 = local write "Q"(w224) -> ()
              }
            }
            n171 = Enqueue Element(queue=w219, element=TD_Input_Quantities_qeue_values."current Q to datain") -> ()  [unwired: 2 in, 3 out]
          }
          frame True {
          }
        }
      }
      event "value-clear": Value Change {
        n172 = event-data() -> ()  [unwired: 1 in, 6 out]
        n173 = flat-sequence {
          tunnel: w250 -> [w252]
          tunnel: [w252] -> w249
          frame #0 {
            n174 = local read "Q"() -> (w255:T2)
            n175 = Bundle By Name(cluster=w255, "Value"=dbl[][] []) -> (w254:T2)
            n176 = local write "Q"(w254) -> ()
          }
        }
        n177 = Enqueue Element(queue=w249, element=TD_Input_Quantities_qeue_values."current Q to datain") -> ()  [unwired: 2 in, 3 out]
      }
      event "uncertainty-clear": Value Change {
        n178 = event-data() -> ()  [unwired: 1 in, 6 out]
        n179 = flat-sequence {
          tunnel: w257 -> [w259]
          tunnel: [w259] -> w256
          frame #0 {
            n180 = local read "Q"() -> (w262:T2)
            n181 = Bundle By Name(cluster=w262, "Uncertainty"=dbl[][] [] ("Value")) -> (w261:T2)
            n182 = local write "Q"(w261) -> ()
          }
        }
        n183 = Enqueue Element(queue=w256, element=TD_Input_Quantities_qeue_values."current Q to datain") -> ()  [unwired: 2 in, 3 out]
      }
      event "dof-clear": Value Change {
        n184 = event-data() -> ()  [unwired: 1 in, 6 out]
        n185 = flat-sequence {
          tunnel: [w266] -> w264
          tunnel: w263 -> [w266]
          frame #0 {
            n186 = local read "Q"() -> (w269:T2)
            n187 = Bundle By Name(cluster=w269, "Degrees of Freedom"=dbl[][] [] ("Value")) -> (w268:T2)
            n188 = local write "Q"(w268) -> ()
          }
        }
        n189 = Enqueue Element(queue=w264, element=TD_Input_Quantities_qeue_values."current Q to datain") -> ()  [unwired: 2 in, 3 out]
      }
      event "corr-clear": Value Change {
        n190 = event-data() -> ()  [unwired: 1 in, 6 out]
        n191 = flat-sequence {
          tunnel: w271 -> [w273]
          tunnel: [w273] -> w270
          frame #0 {
            n192 = local read "Q"() -> (w276:T2)
            n193 = Bundle By Name(cluster=w276, "Correlation"=dbl[][] [] ("Value")) -> (w275:T2)
            n194 = local write "Q"(w275) -> ()
          }
        }
        n195 = Enqueue Element(queue=w270, element=TD_Input_Quantities_qeue_values."current Q to datain") -> ()  [unwired: 2 in, 3 out]
      }
      event "rand-clear": Value Change {
        n196 = event-data() -> ()  [unwired: 1 in, 6 out]
        n197 = flat-sequence {
          tunnel: w278 -> [w280]
          tunnel: [w280] -> w277
          frame #0 {
            n198 = local read "Q"() -> (w283:T2)
            n199 = Bundle By Name(cluster=w283, "Randomized uncertainty"=dbl[][] [] ("Value")) -> (w282:T2)
            n200 = local write "Q"(w282) -> ()
          }
        }
        n201 = Enqueue Element(queue=w277, element=TD_Input_Quantities_qeue_values."current Q to datain") -> ()  [unwired: 2 in, 3 out]
      }
      event "generate wvfrm": Value Change {
        n202 = event-data() -> ()  [unwired: 1 in, 6 out]
        n203 = call "generate wvfrm.vi"() -> ("error out"=w289:errorcluster, "waveform"=w292:dbl[], "time series"=w293:dbl[], "canceled?"=w290:bool)  [unwired: 8 in]
        n204 = Compound Arithmetic op=OR(w290, w289) -> (w288:bool)
        n205 = case shown="False" w288 {
          tunnel: w293 -> [w306 _]
          tunnel: w292 -> [w302 _]
          tunnel: w291 -> [w297 w308]
          tunnel: [w297 w308] -> w284
          frame False {
            w300 = T5 {"Name"="", "Value"=[], "Uncertainty"=[], "Degrees of\nFreedom"=[], "Correlation"=[], "Randomized uncertainty"=[]} ("Quantity")
            n206 = Build Array(w306) -> (w305:dbl[][])
            n207 = Build Array(w302) -> (w301:dbl[][])
            n208 = global read "globals.vi" "Data In"() -> (w307:T2[])
            n209 = Bundle By Name(cluster=w300, "Name"="t", "Value"=w305) -> (w298:T5)
            n210 = Bundle By Name(cluster=w300, "Name"="y", "Value"=w301) -> (w299:T5)
            n211 = Build Array (concatenate)(w307, w298, w299) -> (w294:T2[])
            n212 = global write "globals.vi" "Data In"(w294) -> ()
            n213 = Array Size(array=w294) -> (size(s)=w296:i32)
            n214 = Decrement(x=w296) -> (x-1=w295:i32)
            n215 = local write "current Q index"(w295) -> ()
          }
          frame True {
          }
        }
        n216 = Enqueue Element(queue=w284, element=TD_Input_Quantities_qeue_values."update list of quantities") -> (queue out=w286:refnum<queue>)  [unwired: 2 in, 2 out]
        n217 = Enqueue Element(queue=w286, element=TD_Input_Quantities_qeue_values."show current quantity") -> ()  [unwired: 2 in, 3 out]
      }
    }
  }
